vi "9.2.vi"() -> ()   [LabVIEW 2019]
panel:
  out "kan niet":dbl[](array[numeric])
  out "gedeeld door 3/4/5":dbl[](array[numeric])
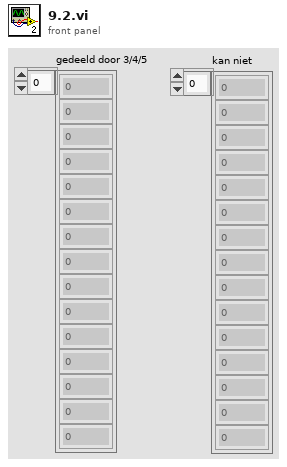
[diagram p1: front panel]
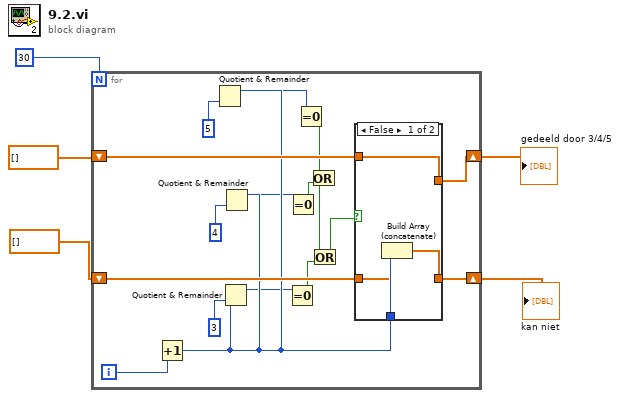
[diagram p0: block diagram]
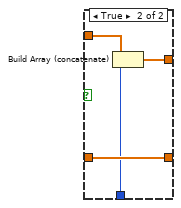
[diagram p2: hidden frame]
diagram:
  n1 = for {
    N: 30 -> [_]
    shift-right: [w17] -> w3
    shift-left: dbl[] [] ("Array") -> [w20]
    shift-right: [w18] -> w2
    shift-left: dbl[] [] ("Array") -> [w19]
    i -> [w21]
    n2 = Increment(x=w21) -> (x+1=w14:i32)
    n3 = Quotient & Remainder(x=w14, y=5) -> (x-y*floor(x/y)=w11:i32)  [unwired: 1 out]
    n4 = Quotient & Remainder(x=w14, y=3) -> (x-y*floor(x/y)=w13:i32)  [unwired: 1 out]
    n5 = Quotient & Remainder(x=w14, y=4) -> (x-y*floor(x/y)=w12:i32)  [unwired: 1 out]
    n6 = Equal To 0?(x=w13) -> (x = 0?=w7:bool)
    n7 = Equal To 0?(x=w12) -> (x = 0?=w9:bool)
    n8 = Equal To 0?(x=w11) -> (x = 0?=w10:bool)
    n9 = Or(x=w10, y=w9) -> (x .or. y?=w8:bool)
    n10 = Or(x=w8, y=w7) -> (x .or. y?=w6:bool)
    n11 = case shown="False" w6 {
      tunnel: w20 -> [w23 w30]
      tunnel: w19 -> [w25 w29]
      tunnel: [w24 w29] -> w18
      tunnel: w14 -> [w26 w28]
      tunnel: [w23 w27] -> w17
      frame False {
        n12 = Build Array (concatenate)(w25, w26) -> (w24:dbl[])
      }
      frame True {
        n13 = Build Array (concatenate)(w30, w28) -> (w27:dbl[])
      }
    }
  }
  "gedeeld door 3/4/5" <- w3
  "kan niet" <- w2
